vi "Q8381 SPAN_START.vi"(1 "unit":u16(ring) items=["um ", "nm"], 2 "value":dbl=1.55 min=0.55 max=17850.0 format="%.4f", 3 "GPIB Address":u16=8 max=31 step=1, 4 "VISA resource name":refnum<visa-resource-name>) -> (0 "Status":bool)   [LabVIEW 2017]
doc: "unit: 0: um 1: nm"
panel:
  out "Program Code":string
  # "SPAN__START"
  # "Precision(um : 4  nm : 1)"
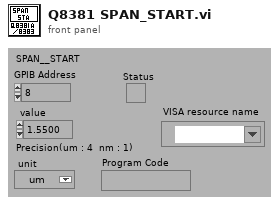
[diagram p1: front panel]
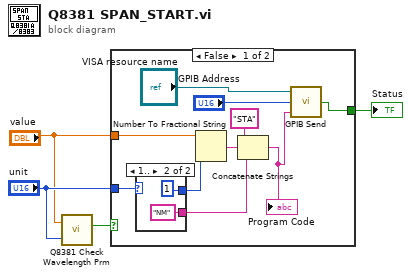
[diagram p0: block diagram]
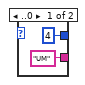
[diagram p2: hidden frame]
diagram:
  n1 = call "Q8381 Check Wavelength Prm.vi"("Unit"="unit", "Wavelength"="value") -> ("GPIB Status"=w2:bool)
  n2 = case shown="False" w2 {
    selector: w2 -> [_ w19]
    tunnel: "unit" -> [w10 _]
    tunnel: "value" -> [w9 _]
    tunnel: [w8 w19] -> w1
    frame False {
      n3 = case shown="1.." w10 {
        tunnel: ["UM" "NM"] -> w12
        tunnel: [4 1] -> w14
        frame ..0 {
        }
        frame 1.. {
        }
      }
      n4 = Number To Fractional String(number=w9, precision (6)=w14) -> (F-format string=w11:string)  [unwired: 2 in]
      n5 = Concatenate Strings("STA", w11, w12) -> (w5:string)
      "Program Code" <- w5
      n6 = call "GPIB Send.vi"("Command String"=w5, "Address"="GPIB Address", "VISA resource name"="VISA resource name") -> ("Error"=w8:bool)
    }
    frame True {
    }
  }
  "Status" <- w1
